vi "ISO 8601 UTC Format String.vi"() -> (1 "ISO 8601 UTC f-string":string="%^<%Y-%m-%dT%H:%M:%S%3uZ>T")   [LabVIEW 2018, in "Utilities.lvlib"]
uses:
  Utilities.lvlib
panel:
  # "Connector Pane"
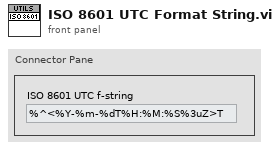
[diagram p1: front panel]
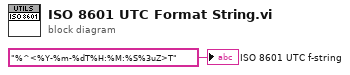
[diagram p0: block diagram]
diagram:
  "ISO 8601 UTC f-string" <- "%^<%Y-%m-%dT%H:%M:%S%3uZ>T"
